vi "Micro-PL Stability Test v10.0.0.vi"() -> ()   [LabVIEW 2010]
uses:
  <vilib>/Utility/miscctls.llb/LVPointTypeDef.ctl
panel:
  in  "Start":bool
  out "Current Time":dbl format="%<%H:%M:%S>t"
  out "Progress":u8(slide) max=10 scale=0.0..100.0
  in  "Total Unit":u16(ring)=2 caption="Unit" items=["s", "min", "h"]
  in  "Total":i32=1 min=1 max=1000 step=1
  in  "Exit":bool
  in  "Interval Unit":u16(ring)=1 caption="Unit" items=["s", "min", "h"]
  in  "Intervall":i32=1 min=0 max=1000 step=1
  # "Stability"
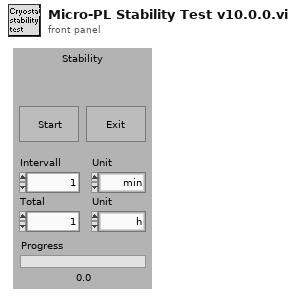
[diagram p1: front panel]
types:
  T1 = typedef "LVPointTypeDef.ctl" = cluster{"Horizontal":i16, "Vertical":i16}
  T2 = enum32{"invalid app kind", "Development System", "Run Time System", "Student Edition", "Embedded LabVIEW", "Evaluation", "Custom"}
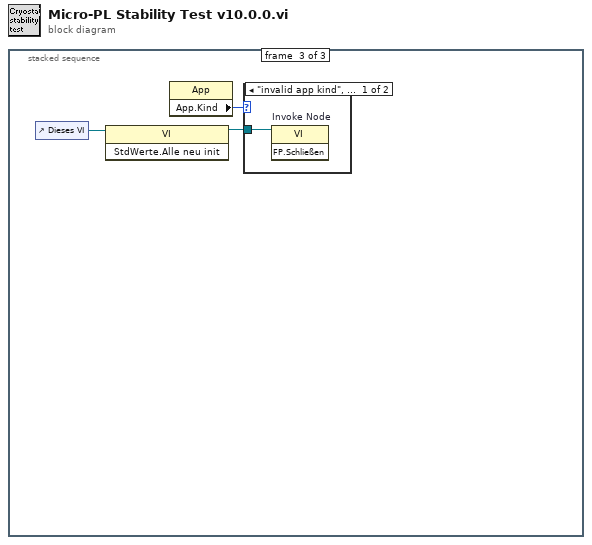
[diagram p0: block diagram]
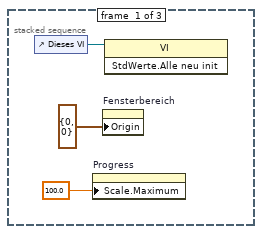
[diagram p2: hidden frame]
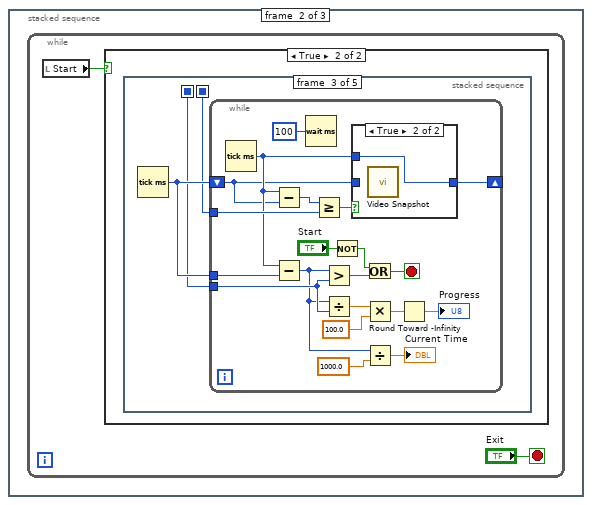
[diagram p3: hidden frame]
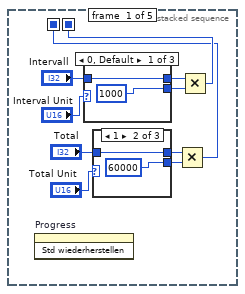
[diagram p5: hidden frame]
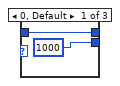
[diagram p6: hidden frame]
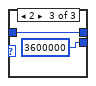
[diagram p7: hidden frame]
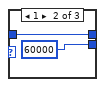
[diagram p8: hidden frame]
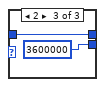
[diagram p9: hidden frame]
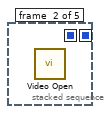
[diagram p10: hidden frame]
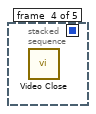
[diagram p12: hidden frame]
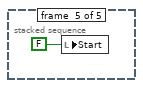
[diagram p13: hidden frame]
diagram:
  n1 = stacked-sequence {
    frame #0 {
      n2 = control-ref of="Dieses VI"() -> (w2:refnum<vi>)
      n3 = property on="Progress" class="Schieber (strikt)"("Scale.Maximum"=100.0 ("Skalierung.Bereich:Maximum")) -> ()  [unwired: 2 in, 2 out]
      n4 = property on="Fensterbereich" class="Bereich"("Origin"=T1 {"Horizontal"=0, "Vertical"=0}) -> ()  [unwired: 2 in, 2 out]
      n5 = invoke class="VI" method="StdWerte.Alle neu init"(reference=w2) -> ()  [unwired: 2 in, 3 out]
    }
    frame #1 {
      n6 = while {
        stop <- "Exit" stop-if-true
        n7 = local read "Start"() -> (w5:bool)
        n8 = case shown="True" w5 {
          frame False {
          }
          frame True {
            n9 = stacked-sequence {
              seq-local: [w7 _ _ _ _] -> [_ _ w29 _ _]
              seq-local: [w6 _ _ _ _] -> [_ _ w28 _ _]
              frame #0 {
                n10 = invoke on="Progress" class="Schieber (strikt)" method="Std wiederherstellen"() -> ()  [unwired: 3 in, 3 out]
                n11 = case shown="0, Default" "Interval Unit" {
                  tunnel: [1000 ("y") 60000 ("y") 3600000 ("y")] -> w15
                  tunnel: "Intervall" -> [w22 w24 w26]
                  tunnel: [w22 w24 w26] -> w12
                  frame 0, Default {
                  }
                  frame 1 {
                  }
                  frame 2 {
                  }
                }
                n12 = case shown="1" "Total Unit" {
                  tunnel: [1000 ("y") 60000 ("y") 3600000 ("y")] -> w11
                  tunnel: "Total" -> [w16 w18 w20]
                  tunnel: [w16 w18 w20] -> w10
                  frame 0, Default {
                  }
                  frame 1 {
                  }
                  frame 2 {
                  }
                }
                n13 = Multiply(x=w10, y=w11) -> (x*y=w6:i32)
                n14 = Multiply(x=w12, y=w15) -> (x*y=w7:i32)
              }
              frame #1 {
                n15 = call "Video Open.vi"() -> ()  [unwired: 11 in, 1 out]
              }
              frame #2 {
                n16 = Tick Count (ms)() -> (millisecond timer value=w30:u32)
                n17 = while {
                  tunnel: w30 -> [w50]
                  shift-right: [w44] -> _
                  shift-left: w30 -> [w41]
                  tunnel: w29 -> [w46]
                  tunnel: w28 -> [w39]
                  stop <- w48 stop-if-true
                  n18 = Tick Count (ms)() -> (millisecond timer value=w42:u32)
                  n19 = Subtract(x=w42, y=w41) -> (x-y=w47:u32)
                  n20 = Subtract(x=w42, y=w50) -> (x-y=w34:u32)
                  n21 = Wait (ms)(milliseconds to wait=u32 100 ("Zu wartende ms")) -> ()  [unwired: 1 out]
                  n22 = Greater Or Equal?(x=w47, y=w46) -> (x >= y?=w45:bool)
                  n23 = Greater?(x=w34, y=w39) -> (0:w49:bool)
                  n24 = Divide(x=w34, y=w39) -> (x/y=w40:dbl)
                  n25 = Not(x="Start") -> (.not. x?=w31:bool)
                  n26 = case shown="True" w45 {
                    tunnel: [w51 w52] -> w44
                    tunnel: w41 -> [w51 _]
                    tunnel: w42 -> [_ w52]
                    frame False {
                    }
                    frame True {
                      n27 = call "Video Snapshot.vi"() -> ()  [unwired: 11 in, 1 out]
                    }
                  }
                  n28 = Or(x=w31, y=w49) -> (x .or. y?=w48:bool)
                  n29 = Multiply(x=w40, y=100.0) -> (x*y=w37:dbl)
                  n30 = Divide(x=w34, y=1000.0) -> (x/y=→"Current Time":dbl)
                  n31 = Round Toward -Infinity(1:w37) -> (0:→"Progress":dbl)
                }
              }
              frame #3 {
                n32 = call "Video Close.vi"() -> ()  [unwired: 11 in, 1 out]
              }
              frame #4 {
                n33 = local write "Start"(FALSE ("Start")) -> ()
              }
            }
          }
        }
      }
    }
    frame #2 {
      n34 = control-ref of="Dieses VI"() -> (w56:refnum<vi>)
      n35 = invoke class="VI" method="StdWerte.Alle neu init"(reference=w56) -> (reference out=w54:refnum<vi>)  [unwired: 2 in, 2 out]
      n36 = property class="App"() -> ("App.Kind"=w55:T2)  [unwired: 2 in, 2 out]
      n37 = case shown="\"invalid app kind\", Default" w55 {
        tunnel: w54 -> [w57 _]
        frame "invalid app kind", Default {
          n38 = invoke on="Invoke Node" class="VI" method="FP.Schließen"(reference=w57) -> ()  [unwired: 2 in, 3 out]
        }
        frame "Development System" {
        }
      }
    }
  }
